vi "Magnetic Drift Correction (1).vi"() -> ()   [LabVIEW 2025]
uses:
  <instrlib>/SMS LabVIEW Drivers/Source Code/Cryogenic Ltd SMSXXX.lvlib
  LabVIEW VI's/Instrument VI's/Instrument Controls/Magnet Array.ctl
  <instrlib>/SMS LabVIEW Drivers/Source Code/Public/PSU Status.ctl
  Labview-File/QMH (STM Auto)/CTL's/Scan_Params (QMH).ctl
  Labview-File/Magnetic Drift Correction/XY_Coords(Final).ctl
panel:
  in  "P-Mode Ramp Rate (A/s)":dbl
  out "Final coordinates (m)":cluster{"Xc":sgl, "Yc":sgl} {"Yc" format="%.4p"; "Xc" format="%.4p"}
  out "Initial coordinates (m)":cluster{"Xc":sgl, "Yc":sgl} {"Yc" format="%.4p"; "Xc" format="%.4p"}
  out "Translation (m)":T1
  out "Output (T)":dbl
  out "MID Setpoint (T)":dbl
  in  "Field Range":T2={"Sweep States"=enum."SET FIELD", "VISA Connection"="COM4", "Fields(T)"=[]}
  in  "Lead- Mode Ramp Rate (A/s)":dbl=0.02
  in  "Start":bool
  out "Errors":errorcluster[](array[cluster])
  in  "stop":bool
  out "Current Index":i32
  in  "Next Field":bool
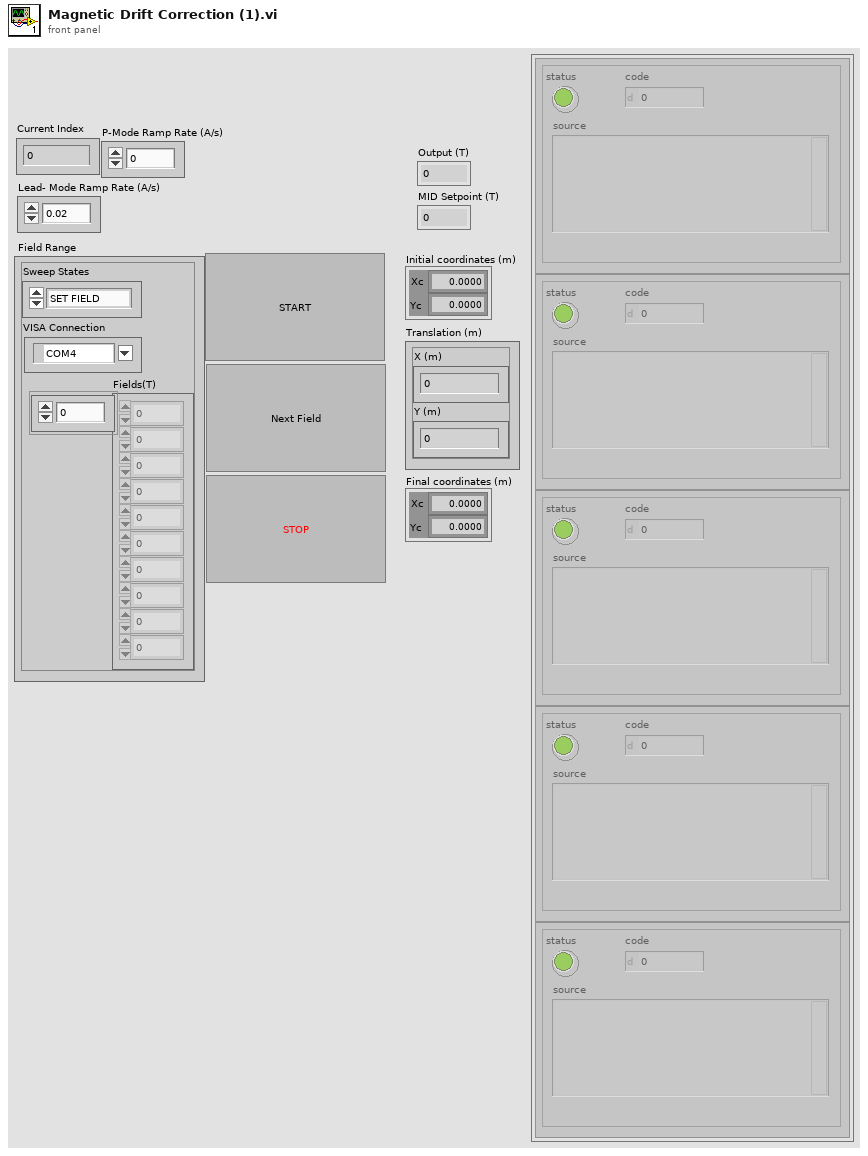
[diagram p1: front panel]
types:
  T1 = typedef "XY_Coords(Final).ctl" = cluster{"X (m)":dbl, "Y (m)":dbl}
  T2 = cluster{"Sweep States":enum16{"SET FIELD", "SWEEP IDLE", "NEXT FIELD", "SWEEP DONE"}, "VISA Connection":refnum<visa-resource-name>, "Fields(T)":dbl[]}
  T3 = enum16{"1. INIT MAG", "2. MAG ON", "3. MAG_STAB", "4. MAG IDLE", "5. PREP NEXT FIELD", "6. APPLY NEXT FIELD", "7. PREP OFF", "8. MAG OFF (Reset)"}
  T4 = typedef "Scan_Params (QMH).ctl" = cluster{"Setpoint (I)":dbl[], "Bias (V)":dbl[], "Number of scans":u8, "Port number (3364)":u32, "Avoid zero threshold (V)":dbl, "Current State":enum16{"1. BIAS", "2. INIT_SCAN", "3. SCAN_IDLE", "4. INTER_SCAN", "5. NEW_COORDS_&_FRAME", "6. FINAL_SCAN", "7. POLL BIAS", "8. Z-CONT", "9. STOP"}}
  T5 = enum16{"1. BIAS", "2. INIT_SCAN", "3. SCAN_IDLE", "4. INTER_SCAN", "5. NEW_COORDS_&_FRAME", "6. FINAL_SCAN", "7. STOP"}
  T6 = typedef "Cryogenic Ltd SMSXXX.lvlib/PSU Status.ctl" = cluster{"Ramp Target":enum16{"ZERO", "MID", "MAX"}, "Pause":bool, "Switch Heater":bool, "Persistent Field":dbl, "Persistent Current":dbl, "Tesla":bool, "Output (T)":dbl, "Output (A)":dbl, "X Trip":enum16{"DISABLED", "ENABLED", "ACTIVE"}, "Ramp Rate (A/s)":dbl, "V Limit (V)":dbl, "Heater Voltage":dbl, "MAX Setpoint (A)":dbl, "MAX Setpoint (T)":dbl, "MID Setpoint (A)":dbl, "MID Setpoint (T)":dbl, "Lock":bool, "Field Constant":dbl, "Remote":bool, "Direction":enum16{"POSITIVE", "NEGATIVE", "OPEN", "UNIPOLAR"}, "Helium Level":u16, "Quench !":bool, "Voltage":dbl, "V Limit !":bool, "Ramping":bool, "At Target":bool, "Trip Field":dbl, "Trip Current":dbl, "Enum":enum16{"1. INIT MAG", "2. MAG ON ", "3. MAG_STAB", "4. MAG IDLE", "5. NEXT FIELD", "6. MAG OFF (Reset)"}}
  T7 = enum16{"SET FIELD", "SWEEP IDLE", "NEXT FIELD", "SWEEP DONE"}
  T8 = typedef "Magnet Array.ctl" = cluster{"Sweep States":enum16{"SET FIELD", "SWEEP IDLE", "NEXT FIELD", "SWEEP DONE"}, "VISA Connection":refnum<visa-resource-name>, "Fields(T)":dbl[]}
  T9 = typedef "Scan_Params (QMH).ctl" = cluster{"Setpoint (I)":dbl[], "Bias (V)":dbl[], "Number of scans":u8, "Port number (3364)":u32, "Avoid zero threshold (V)":dbl, "Current State":enum16{"1. BIAS", "2. INIT_SCAN", "3. SCAN_IDLE", "4. INTER_SCAN", "5. NEW_COORDS_&_FRAME", "6. FINAL_SCAN", "7. POLL BIAS ", "8. STOP"}}
  T10 = enum16{"1. BIAS", "2. INIT_SCAN", "3. SCAN_IDLE", "4. INTER_SCAN", "5. NEW_COORDS_&_FRAME", "6. FINAL_SCAN", "7. POLL BIAS ", "8. STOP"}
  T11 = typedef "Bias Cont QMH.ctl" = cluster{"Machine name (local machine IP)":string, "Port number (3364)":u32, "Current State":enum16{"Bias", "Stop"}, "Inital X (m)":dbl, "Initial Y (m)":dbl, "Final X (m)":sgl, "Final Y (m)":sgl}
  T12 = enum16{"RAMP TO ZERO", "RAMP TO MID", "RAMP TO MAX"}
  T13 = typedef "PSU Status.ctl" = cluster{"Ramp Target":enum16{"ZERO", "MID", "MAX"}, "Pause":bool, "Switch Heater":bool, "Persistent Field":dbl, "Persistent Current":dbl, "Tesla":bool, "Output (T)":dbl, "Output (A)":dbl, "X Trip":enum16{"DISABLED", "ENABLED", "ACTIVE"}, "Ramp Rate (A/s)":dbl, "V Limit (V)":dbl, "Heater Voltage":dbl, "MAX Setpoint (A)":dbl, "MAX Setpoint (T)":dbl, "MID Setpoint (A)":dbl, "MID Setpoint (T)":dbl, "Lock":bool, "Field Constant":dbl, "Remote":bool, "Direction":enum16{"POSITIVE", "NEGATIVE", "OPEN", "UNIPOLAR"}, "Helium Level":u16, "Quench !":bool, "Voltage":dbl, "V Limit !":bool, "Ramping":bool, "At Target":bool, "Trip Field":dbl, "Trip Current":dbl, "Current State":enum16{"1. INIT MAG", "2. MAG ON", "3. MAG_STAB", "4. MAG IDLE", "5. PREP NEXT FIELD", "6. APPLY NEXT FIELD", "7. PREP OFF", "8. MAG OFF (Reset)"}, "MAG Reference":refnum<visa-resource-name>}
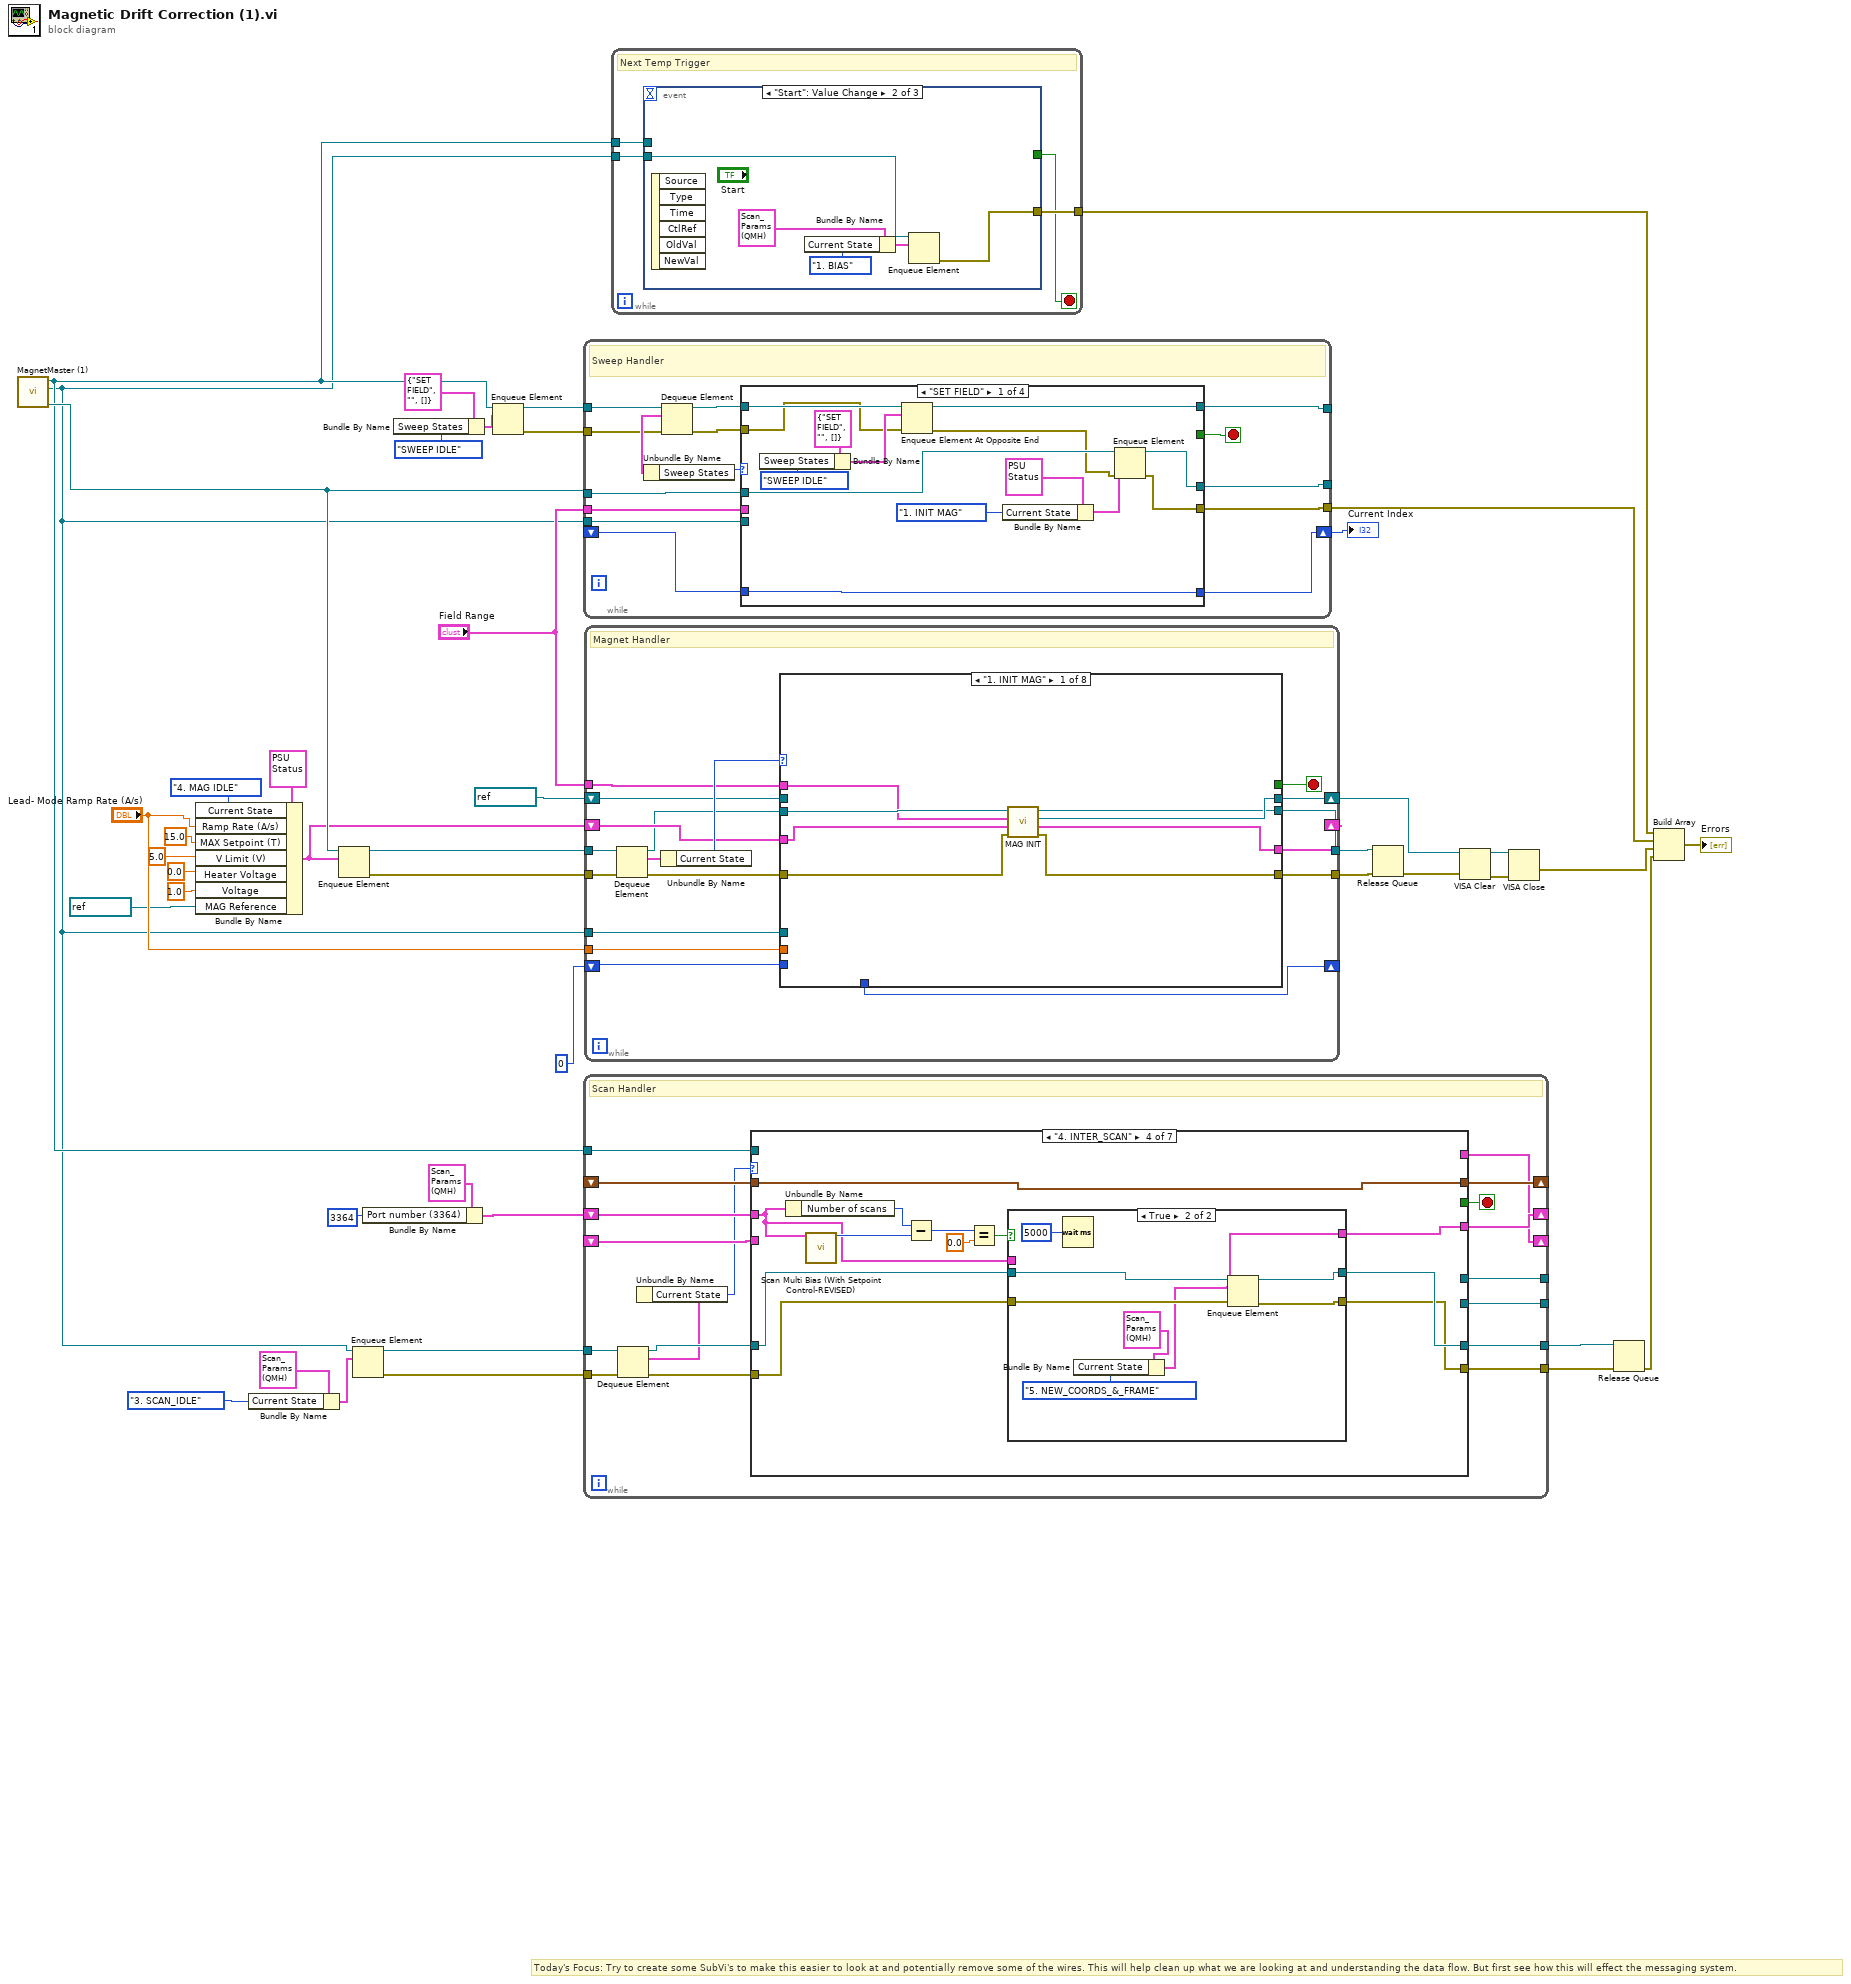
[diagram p0: block diagram]
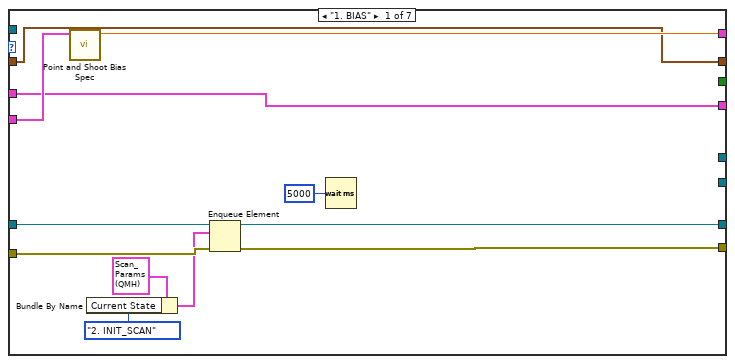
[diagram p2: hidden frame]
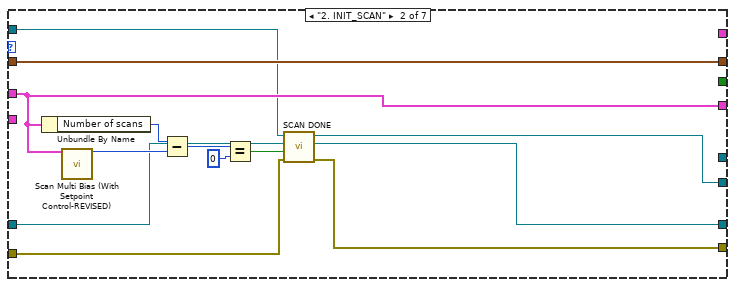
[diagram p3: hidden frame]
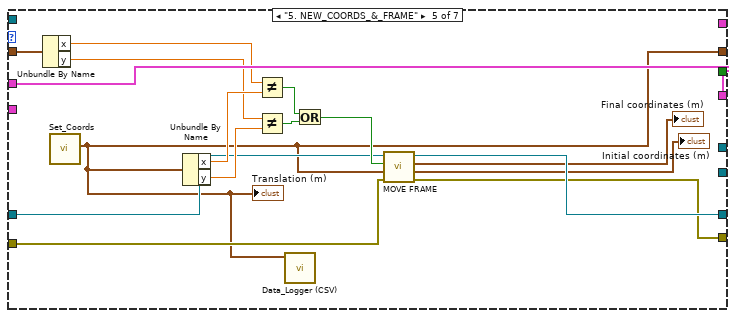
[diagram p6: hidden frame]
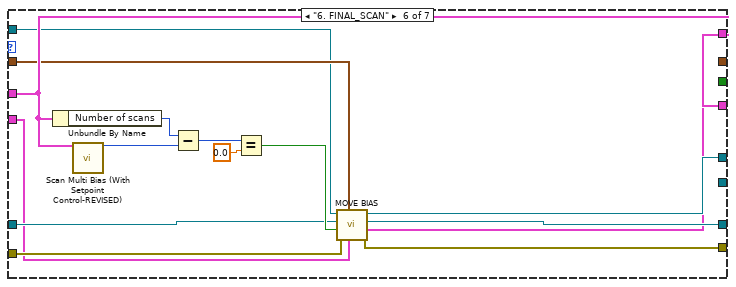
[diagram p7: hidden frame]
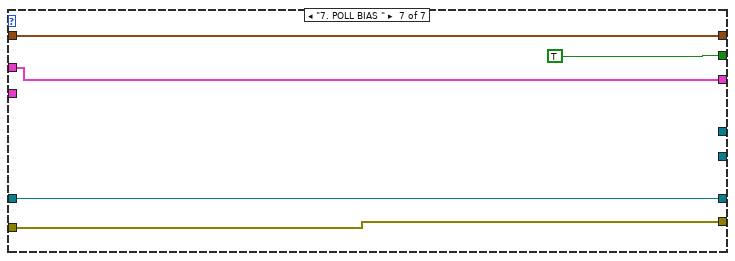
[diagram p8: hidden frame]
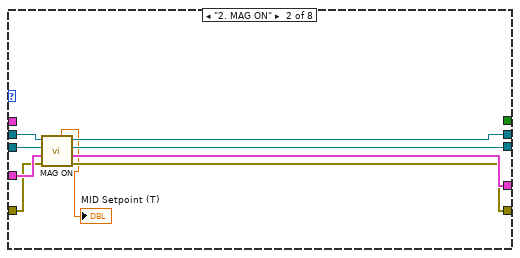
[diagram p9: hidden frame]
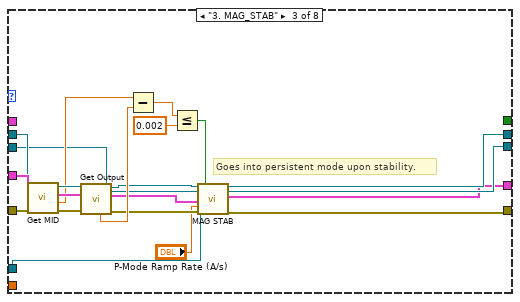
[diagram p10: hidden frame]
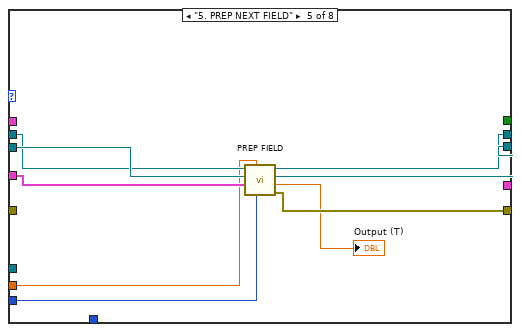
[diagram p12: hidden frame]
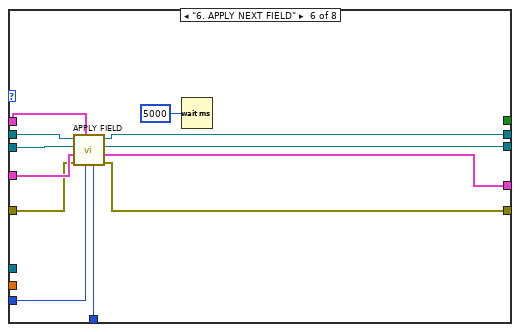
[diagram p13: hidden frame]
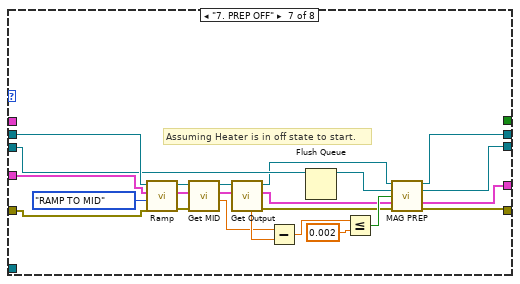
[diagram p14: hidden frame]
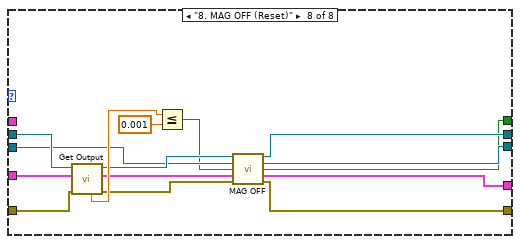
[diagram p15: hidden frame]
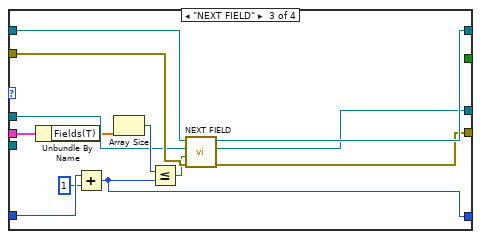
[diagram p17: hidden frame]
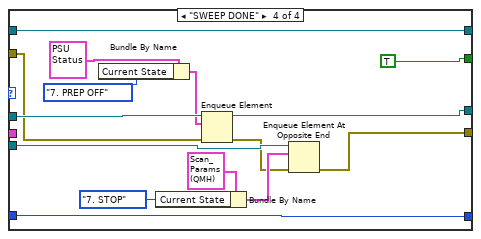
[diagram p18: hidden frame]
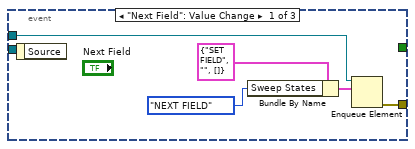
[diagram p19: hidden frame]
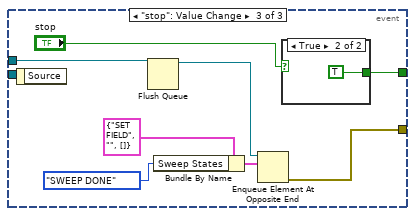
[diagram p20: hidden frame]
diagram:
  # "Today's Focus: Try to create some SubVi's to make this easier to look at and potentially remove some of the wires. This will help clean up what we are looking at and understanding the data flow. But first see how this will effect the messaging system."
  n1 = call "MagnetMaster (1).vi"() -> ("MagQ"=w34:refnum<queue>, "ScanQ"=w1:refnum<queue>, "SweepQ"=w2:refnum<queue>)  [unwired: 9 in]
  n2 = Bundle By Name(cluster=T6 {"Ramp Target"=enum."ZERO", "Pause"=FALSE, "Switch Heater"=FALSE, "Persistent Field"=0.0, "Persistent Current"=0.0, "Tesla"=FALSE, "Output (T)"=0.0, "Output (A)"=0.0, "X Trip"=enum."DISABLED", "Ramp Rate (A/s)"=0.0, "V Limit (V)"=0.0, "Heater Voltage"=0.0, "MAX Setpoint (A)"=0.0, "MAX Setpoint (T)"=0.0, "MID Setpoint (A)"=0.0, "MID Setpoint (T)"=0.0, "Lock"=FALSE, "Field Constant"=0.0, "Remote"=FALSE, "Direction"=enum."POSITIVE", "Helium Level"=0, "Quench !"=FALSE, "Voltage"=0.0, "V Limit !"=FALSE, "Ramping"=FALSE, "At Target"=FALSE, "Trip Field"=0.0, "Trip Current"=0.0, "Enum"=enum."1. INIT MAG"} ("PSU Status In"), "Current State"=T3."4. MAG IDLE", "Ramp Rate (A/s)"="Lead- Mode Ramp Rate (A/s)", "MAX Setpoint (T)"=15.0, "V Limit (V)"=5.0, "Heater Voltage"=0.0, "Voltage"=1.0, "MAG Reference"=refnum<visa-resource-name> "COM4") -> (w30:T6)
  n3 = Bundle By Name(cluster=T4 {"Setpoint (I)"=[], "Bias (V)"=[], "Number of scans"=1, "Port number (3364)"=3364, "Avoid zero threshold (V)"=0.004999999888241291, "Current State"=enum."1. BIAS"} ("element"), "Current State"=T5."3. SCAN_IDLE") -> (w19:T4)
  n4 = Enqueue Element(queue=w34, element=w30) -> (queue out=w33:refnum<queue>, error out=w32:errorcluster)  [unwired: 2 in, 1 out]
  n5 = Enqueue Element(queue=w1, element=w19) -> (queue out=w21:refnum<queue>, error out=w20:errorcluster)  [unwired: 2 in, 1 out]
  n6 = Bundle By Name(cluster=T4 {"Setpoint (I)"=[], "Bias (V)"=[], "Number of scans"=1, "Port number (3364)"=3364, "Avoid zero threshold (V)"=0.004999999888241291, "Current State"=enum."1. BIAS"} ("element"), "Port number (3364)"=u32 3364) -> (w12:T4)
  n7 = Bundle By Name(cluster=T8 {"Sweep States"=enum."SET FIELD", "VISA Connection"="", "Fields(T)"=[]} ("element"), "Sweep States"=T7."SWEEP IDLE") -> (w37:T8)
  n8 = Enqueue Element(queue=w2, element=w37) -> (queue out=w39:refnum<queue>, error out=w35:errorcluster)  [unwired: 2 in, 1 out]
  n9 = while {
    tunnel: w39 -> [w58]
    shift-right: [w53] -> w44
    shift-left: _ -> [w56]
    tunnel: [w55] -> _
    tunnel: [w52] -> _
    tunnel: [w50] -> w28
    tunnel: w34 -> [w48]
    tunnel: w35 -> [w47]
    tunnel: "Field Range" -> [w46]
    tunnel: w1 -> [w45]
    stop <- w49 stop-if-true
    # "Sweep Handler"
    n10 = Dequeue Element(queue=w58, error in (no error)=w47) -> (queue out=w54:refnum<queue>, element=w57:T8, error out=w51:errorcluster)  [unwired: 1 in, 1 out]
    n11 = Unbundle By Name(w57) -> ("Sweep States"=w59:T7)
    n12 = case shown="\"SET FIELD\"" w59 {
      tunnel: w56 -> [w72 _ w86 w100]
      tunnel: [w73 _ w77 w96] -> w55
      tunnel: w54 -> [w71 _ w83 w101]
      tunnel: [w72 _ w76 w100] -> w53
      tunnel: [w70 _ w82 w101] -> w52
      tunnel: w51 -> [w65 _ w81 w97]
      tunnel: [w63 _ w80 w87] -> w50
      tunnel: [_ _ _ TRUE] -> w49
      tunnel: w48 -> [w69 _ w78 w98]
      tunnel: w46 -> [_ _ w74 _]
      tunnel: w45 -> [_ _ _ w91]
      frame "SET FIELD" {
        n13 = Bundle By Name(cluster=T8 {"Sweep States"=enum."SET FIELD", "VISA Connection"="", "Fields(T)"=[]} ("element"), "Sweep States"=T7."SWEEP IDLE") -> (w67:T8)
        n14 = Enqueue Element At Opposite End(queue=w71, element=w67, error in (no error)=w65) -> (queue out=w70:refnum<queue>, error out=w64:errorcluster)  [unwired: 1 in, 1 out]
        n15 = Bundle By Name(cluster=T6 {"Ramp Target"=enum."ZERO", "Pause"=FALSE, "Switch Heater"=FALSE, "Persistent Field"=0.0, "Persistent Current"=0.0, "Tesla"=FALSE, "Output (T)"=0.0, "Output (A)"=0.0, "X Trip"=enum."DISABLED", "Ramp Rate (A/s)"=0.0, "V Limit (V)"=0.0, "Heater Voltage"=0.0, "MAX Setpoint (A)"=0.0, "MAX Setpoint (T)"=0.0, "MID Setpoint (A)"=0.0, "MID Setpoint (T)"=0.0, "Lock"=FALSE, "Field Constant"=0.0, "Remote"=FALSE, "Direction"=enum."POSITIVE", "Helium Level"=0, "Quench !"=FALSE, "Voltage"=0.0, "V Limit !"=FALSE, "Ramping"=FALSE, "At Target"=FALSE, "Trip Field"=0.0, "Trip Current"=0.0, "Enum"=enum."1. INIT MAG"} ("PSU Status In"), "Current State"=T3."1. INIT MAG") -> (w61:T6)
        n16 = Enqueue Element(queue=w69, element=w61, error in (no error)=w64) -> (queue out=w73:refnum<queue>, error out=w63:errorcluster)  [unwired: 1 in, 1 out]
      }
      frame "SWEEP IDLE" {
      }
      frame "NEXT FIELD" {
        n17 = Unbundle By Name(w74) -> ("Fields(T)"=w75:dbl[])
        n18 = Add(x=w86, y=1) -> (x+y=w76:i32)
        n19 = Array Size(array=w75) -> (size(s)=w84:i32)
        n20 = Less Or Equal?(x=w84, y=w76) -> (x <= y?=w79:bool)
        n21 = call "NEXT FIELD.vi"("error in (no error)"=w81, "Boolean"=w79, "MagQ in"=w78, "Queue in"=w83) -> ("error out"=w80:errorcluster, "MagQ out"=w77:refnum<queue>, "Queue out"=w82:refnum<queue>)  [unwired: 5 in]
      }
      frame "SWEEP DONE" {
        n22 = Bundle By Name(cluster=T6 {"Ramp Target"=enum."ZERO", "Pause"=FALSE, "Switch Heater"=FALSE, "Persistent Field"=0.0, "Persistent Current"=0.0, "Tesla"=FALSE, "Output (T)"=0.0, "Output (A)"=0.0, "X Trip"=enum."DISABLED", "Ramp Rate (A/s)"=0.0, "V Limit (V)"=0.0, "Heater Voltage"=0.0, "MAX Setpoint (A)"=0.0, "MAX Setpoint (T)"=0.0, "MID Setpoint (A)"=0.0, "MID Setpoint (T)"=0.0, "Lock"=FALSE, "Field Constant"=0.0, "Remote"=FALSE, "Direction"=enum."POSITIVE", "Helium Level"=0, "Quench !"=FALSE, "Voltage"=0.0, "V Limit !"=FALSE, "Ramping"=FALSE, "At Target"=FALSE, "Trip Field"=0.0, "Trip Current"=0.0, "Enum"=enum."1. INIT MAG"} ("PSU Status In"), "Current State"=T3."7. PREP OFF") -> (w94:T6)
        n23 = Bundle By Name(cluster=T4 {"Setpoint (I)"=[], "Bias (V)"=[], "Number of scans"=1, "Port number (3364)"=3364, "Avoid zero threshold (V)"=0.004999999888241291, "Current State"=enum."1. BIAS"} ("element"), "Current State"=T5."7. STOP") -> (w90:T4)
        n24 = Enqueue Element(queue=w98, element=w94, error in (no error)=w97) -> (queue out=w96:refnum<queue>, error out=w88:errorcluster)  [unwired: 1 in, 1 out]
        n25 = Enqueue Element At Opposite End(queue=w91, element=w90, error in (no error)=w88) -> (error out=w87:errorcluster)  [unwired: 1 in, 2 out]
      }
    }
  }
  "Current Index" <- w44
  n26 = while {
    tunnel: w20 -> [w111]
    shift-right: [w116] -> _
    shift-left: w12 -> [w119]
    tunnel: [w118] -> w16
    shift-right: [w115] -> _
    shift-left: _ -> [w114]
    tunnel: [w112] -> w15
    tunnel: [w109] -> _
    shift-right: [w107] -> _
    shift-left: _ -> [w108]
    tunnel: w21 -> [w106]
    tunnel: w2 -> [w105]
    tunnel: [w104] -> _
    stop <- w113 stop-if-true
    # "Scan Handler"
    n27 = Dequeue Element(queue=w106, error in (no error)=w111) -> (queue out=w117:refnum<queue>, element=w102:T9, error out=w110:errorcluster)  [unwired: 1 in, 1 out]
    n28 = Unbundle By Name(w102) -> ("Current State"=w103:T10)
    n29 = case shown="\"4. INTER_SCAN\"" w103 {
      tunnel: w119 -> [w127 w137 w146 w151 w186 w197 w203]
      tunnel: [w128 w138 w145 w153 w177 w193 w205] -> w118
      tunnel: w110 -> [w123 w140 _ w148 w174 w191 w204]
      tunnel: w117 -> [w129 w139 w145 w154 w178 w195 w205]
      tunnel: [w127 w137 w146 w152 w186 w197 w203] -> w116
      tunnel: [w126 w135 w147 w150 w171 _ w202] -> w115
      tunnel: w114 -> [w126 w135 w147 w150 w176 w194 w202]
      tunnel: [_ _ _ _ _ _ TRUE] -> w113
      tunnel: [w124 w134 _ w149 w175 w192 w204] -> w112
      tunnel: [_ _ _ _ _ w190 _] -> w109
      tunnel: w108 -> [w131 _ _ _ _ w188 _]
      tunnel: [w130 _ _ _ _ w189 _] -> w107
      tunnel: w105 -> [_ w133 _ _ _ w187 _]
      tunnel: [_ w132 _ _ _ _ _] -> w104
      frame "1. BIAS" {
        n30 = call "Point and Shoot Bias Spec.vi"("Bias Controller"=w131) -> ("Inital X (m)"=w130:dbl)  [unwired: 9 in, 1 out]
        n31 = Bundle By Name(cluster=T4 {"Setpoint (I)"=[], "Bias (V)"=[], "Number of scans"=1, "Port number (3364)"=3364, "Avoid zero threshold (V)"=0.004999999888241291, "Current State"=enum."1. BIAS"} ("element"), "Current State"=T5."2. INIT_SCAN") -> (w120:T4)
        n32 = Enqueue Element(queue=w129, element=w120, error in (no error)=w123) -> (queue out=w128:refnum<queue>, error out=w124:errorcluster)  [unwired: 1 in, 1 out]
        n33 = Wait (ms)(milliseconds to wait=u32 5000) -> ()  [unwired: 1 out]
      }
      frame "2. INIT_SCAN" {
        n34 = Unbundle By Name(w137) -> ("Number of scans"=w136:u8)
        n35 = call "Scan Multi Bias (With Setpoint Control-REVISED).vi"("Scan Parameters"=w137) -> ("Scan"=w141:u8)  [unwired: 13 in, 1 out]
        n36 = Subtract(x=w136, y=w141) -> (x-y=w144:u8)
        n37 = Equal?(x=w144, y=u8 0) -> (x = y?=w142:bool)
        n38 = call "SCAN DONE.vi"("error in (no error)"=w140, "Boolean"=w142, "ScanQ in"=w139, "Queue in"=w133) -> ("error out"=w134:errorcluster, "ScanQ out"=w138:refnum<queue>, "Queue out"=w132:refnum<queue>)  [unwired: 5 in]
      }
      frame "3. SCAN_IDLE" {
      }
      frame "4. INTER_SCAN" {
        n39 = Unbundle By Name(w151) -> ("Number of scans"=w155:u8)
        n40 = call "Scan Multi Bias (With Setpoint Control-REVISED).vi"("Scan Parameters"=w151) -> ("Scan"=w156:u8)  [unwired: 13 in, 1 out]
        n41 = Subtract(x=w155, y=w156) -> (x-y=w158:u8)
        n42 = Equal?(x=w158, y=0.0) -> (x = y?=w157:bool)
        n43 = case shown="True" w157 {
          tunnel: w154 -> [w162 w169]
          tunnel: [w162 w168] -> w153
          tunnel: [w161 w163] -> w152
          tunnel: w151 -> [w161 _]
          tunnel: [w160 w167] -> w149
          tunnel: w148 -> [w160 w166]
          frame False {
          }
          frame True {
            n44 = Wait (ms)(milliseconds to wait=u32 5000) -> ()  [unwired: 1 out]
            n45 = Bundle By Name(cluster=T4 {"Setpoint (I)"=[], "Bias (V)"=[], "Number of scans"=1, "Port number (3364)"=3364, "Avoid zero threshold (V)"=0.004999999888241291, "Current State"=enum."2. INIT_SCAN"} ("element"), "Current State"=T5."5. NEW_COORDS_&_FRAME") -> (w163:T4)
            n46 = Enqueue Element(queue=w169, element=w163, error in (no error)=w166) -> (queue out=w168:refnum<queue>, error out=w167:errorcluster)  [unwired: 1 in, 1 out]
          }
        }
      }
      frame "5. NEW_COORDS_&_FRAME" {
        n47 = Unbundle By Name(w176) -> ("x"=w180:dbl, "y"=w179:dbl)
        n48 = call "Set_Coords.vi"() -> ("return value"=w171:cluster{"x":dbl, "y":dbl})  [unwired: 10 in, 1 out]
        "Translation (m)" <- w171
        n49 = Unbundle By Name(w171) -> ("x"=w183:dbl, "y"=w182:dbl)
        n50 = Not Equal?(x=w180, y=w183) -> (x != y?=w185:bool)
        n51 = Not Equal?(x=w179, y=w182) -> (x != y?=w184:bool)
        n52 = call "Data_Logger (CSV).vi"("Translation (m)"=w171) -> ()  [unwired: 11 in]
        n53 = Or(x=w185, y=w184) -> (x .or. y?=w181:bool)
        n54 = call "MOVE FRAME.vi"("error in (no error)"=w174, "return value"=w171, "Boolean"=w181, "Queue in"=w178) -> ("error out"=w175:errorcluster, "Initial coordinates (m)"=→"Initial coordinates (m)":cluster{"Xc":sgl, "Yc":sgl}, "Final coordinates (m)"=→"Final coordinates (m)":cluster{"Xc":sgl, "Yc":sgl}, "Queue out"=w177:refnum<queue>)  [unwired: 4 in]
      }
      frame "6. FINAL_SCAN" {
        n55 = Unbundle By Name(w197) -> ("Number of scans"=w196:u8)
        n56 = call "Scan Multi Bias (With Setpoint Control-REVISED).vi"("Scan Parameters"=w197) -> ("Scan"=w199:u8)  [unwired: 13 in, 1 out]
        n57 = Subtract(x=w196, y=w199) -> (x-y=w200:u8)
        n58 = Equal?(x=w200, y=0.0) -> (x = y?=w198:bool)
        n59 = call "MOVE BIAS.vi"("Bias in"=w188, "return value"=w194, "error in (no error)"=w191, "Boolean"=w198, "ScanQ in"=w195, "Queue in"=w187) -> ("error out"=w192:errorcluster, "Bias out 2"=w189:T11, "ScanQ out"=w193:refnum<queue>, "Queue out"=w190:refnum<queue>)  [unwired: 2 in]
      }
      frame "7. POLL BIAS " {
      }
    }
  }
  n60 = while {
    tunnel: w33 -> [w223]
    tunnel: [w219] -> w42
    shift-right: [w218] -> _
    shift-left: w30 -> [w221]
    shift-right: [w217] -> w8
    shift-left: refnum<visa-resource-name> "COM4" ("MAG Reference") -> [w216]
    tunnel: [w215] -> w43
    tunnel: w32 -> [w214]
    tunnel: "Field Range" -> [w213]
    shift-right: [w208] -> _
    shift-left: 0 -> [w212]
    tunnel: "Lead- Mode Ramp Rate (A/s)" -> [w210]
    tunnel: w1 -> [w209]
    stop <- w207 stop-if-true
    # "Magnet Handler"
    n61 = Dequeue Element(queue=w223, error in (no error)=w214) -> (queue out=w211:refnum<queue>, element=w224:T13, error out=w220:errorcluster)  [unwired: 1 in, 1 out]
    n62 = Unbundle By Name(w224) -> ("Current State"=w222:T3)
    n63 = case "MAG STATE MACHINE" shown="\"1. INIT MAG\"" w222 {
      tunnel: w221 -> [w228 w241 w261 w266 w272 w283 w308 w323]
      tunnel: w220 -> [w226 w239 w262 w265 _ w282 w307 w324]
      tunnel: [w231 w236 w242 w265 w269 w286 w288 w311] -> w219
      tunnel: [w229 w237 w243 w266 _ w278 w289 w314] -> w218
      tunnel: [w232 w238 w246 w264 w268 w279 w291 w315] -> w217
      tunnel: w216 -> [_ w240 w260 w264 w271 w284 w309 w325]
      tunnel: [w230 w235 w247 w263 w274 w287 w290 w313] -> w215
      tunnel: w213 -> [w225 _ _ _ _ w281 _ _]
      tunnel: w212 -> [_ _ _ _ w275 w280 _ _]
      tunnel: w211 -> [w227 w234 w251 w263 w273 w277 w299 w318]
      tunnel: w210 -> [_ _ _ _ w270 _ _ _]
      tunnel: w209 -> [_ _ w250 _ _ _ _ _]
      tunnel: [_ _ _ _ _ w276 _ _] -> w208
      tunnel: [_ _ _ _ _ _ _ w312] -> w207
      frame "1. INIT MAG" {
        n64 = call "MAG INIT.vi"("error in (no error)"=w226, "PSU Status In"=w228, "Field and Temp Range"=w225, "Queue in"=w227) -> ("error out"=w231:errorcluster, "PSU Status Out"=w229:T6, "VISA Resource Name Out"=w232:refnum<visa-resource-name>, "Queue out"=w230:refnum<queue>)  [unwired: 4 in]
      }
      frame "2. MAG ON" {
        n65 = call "MAG ON.vi"("error in (no error)"=w239, "PSU Status In"=w241, "MagQ in"=w234, "VISA Refnum in"=w240) -> ("error out"=w236:errorcluster, "PSU Status Out"=w237:T6, "MagQ out"=w235:refnum<queue>, "VISA Refnum out"=w238:refnum<visa-resource-name>, "MID Setpoint (T)"=→"MID Setpoint (T)":dbl)  [unwired: 3 in]
      }
      frame "3. MAG_STAB" {
        # "Goes into persistent mode upon stability."
        n66 = call <instrlib>:"Get MID.vi"("Error in (no error)"=w262, "PSU Status In"=w261, "VISA Resource Name In"=w260) -> ("Error out"=w259:errorcluster, "MID Setpoint (T)"=w255:dbl, "PSU Status Out"=w258:T6, "VISA Resource Name Out"=w257:refnum<visa-resource-name>)  [unwired: 3 in, 2 out]
        n67 = call <instrlib>:"Get Output.vi"("Error in (no error)"=w259, "PSU Status In"=w258, "VISA Resource Name In"=w257) -> ("Error out"=w248:errorcluster, "PSU Status Out"=w249:T6, "VISA Resource Name Out"=w252:refnum<visa-resource-name>, "Output (T)"=w253:dbl)  [unwired: 3 in, 2 out]
        n68 = Subtract(x=w255, y=w253) -> (x-y=w254:dbl)
        n69 = Less Or Equal?(x=w254, y=0.002) -> (x <= y?=w245:bool)
        n70 = call "MAG STAB.vi"("VISA In"=w252, "MagQ"=w251, "ScanQ"=w250, "PSU Status In"=w249, "P-Mode Ramp Rate (A/s)"="P-Mode Ramp Rate (A/s)", "Error out"=w248, "Boolean"=w245) -> ("VISA Out"=w246:refnum<visa-resource-name>, "MagQ"=w247:refnum<queue>, "PSU Status Out"=w243:T6, "error out"=w242:errorcluster)  [unwired: 9 in]
      }
      frame "4. MAG IDLE" {
      }
      frame "5. PREP NEXT FIELD" {
        n71 = call "PREP FIELD.vi"("Numeric"=w275, "Lead- Mode Ramp Rate (A/s)"=w270, "PSU Status In"=w272, "MagQ in"=w273, "VISA Refnum in"=w271) -> ("error out"=w269:errorcluster, "Output (T)"=→"Output (T)":dbl, "MagQ out"=w274:refnum<queue>, "VISA Refnum out"=w268:refnum<visa-resource-name>)  [unwired: 3 in]
      }
      frame "6. APPLY NEXT FIELD" {
        n72 = call "APPLY FIELD.vi"("Numeric in"=w280, "Field and Tep  Range"=w281, "error in (no error)"=w282, "PSU Status In"=w283, "MagQ in"=w277, "VISA Refnum in"=w284) -> ("error out"=w286:errorcluster, "PSU Status Out"=w278:T6, "MagQ out"=w287:refnum<queue>, "VISA Refnum out"=w279:refnum<visa-resource-name>, "Numeric out"=w276:i32)  [unwired: 1 in]
        n73 = Wait (ms)(milliseconds to wait=u32 5000) -> ()  [unwired: 1 out]
      }
      frame "7. PREP OFF" {
        # "Assuming Heater is in off state to start."
        n74 = call <instrlib>:"Ramp.vi"("Error in (no error)"=w307, "Ramp Target"=T12."RAMP TO MID", "PSU Status In"=w308, "VISA Resource Name In"=w309) -> ("Error out"=w304:errorcluster, "PSU Status Out"=w305:T6, "VISA Resource Name Out"=w306:refnum<visa-resource-name>)  [unwired: 4 in, 1 out]
        n75 = call <instrlib>:"Get MID.vi"("Error in (no error)"=w304, "PSU Status In"=w305, "VISA Resource Name In"=w306) -> ("MID Setpoint (T)"=w297:dbl, "PSU Status Out"=w302:T6, "VISA Resource Name Out"=w303:refnum<visa-resource-name>)  [unwired: 3 in, 3 out]
        n76 = call <instrlib>:"Get Output.vi"("PSU Status In"=w302, "VISA Resource Name In"=w303) -> ("Error out"=w292:errorcluster, "PSU Status Out"=w293:T6, "VISA Resource Name Out"=w295:refnum<visa-resource-name>, "Output (T)"=w298:dbl)  [unwired: 4 in, 2 out]
        n77 = Subtract(x=w297, y=w298) -> (x-y=w301:dbl)
        n78 = Flush Queue(queue=w299) -> (queue out=w296:refnum<queue>)  [unwired: 1 in, 2 out]
        n79 = Less Or Equal?(x=w301, y=0.002) -> (x <= y?=w294:bool)
        n80 = call "MAG PREP.vi"("VISA In"=w295, "MagQ"=w296, "Boolean"=w294, "PSU Status In"=w293, "Error In"=w292) -> ("VISA Out"=w291:refnum<visa-resource-name>, "MagQ"=w290:refnum<queue>, "PSU Status Out"=w289:T6, "error out"=w288:errorcluster)  [unwired: 7 in]
      }
      frame "8. MAG OFF (Reset)" {
        n81 = call <instrlib>:"Get Output.vi"("Error in (no error)"=w324, "PSU Status In"=w323, "VISA Resource Name In"=w325) -> ("Error out"=w317:errorcluster, "PSU Status Out"=w319:T6, "VISA Resource Name Out"=w320:refnum<visa-resource-name>, "Output (T)"=w322:dbl)  [unwired: 3 in, 2 out]
        n82 = Less Or Equal?(x=w322, y=0.001) -> (x <= y?=w316:bool)
        n83 = call "MAG OFF.vi"("VISA Resource Name Out"=w320, "MagQ"=w318, "Boolean"=w316, "PSU Status Out"=w319, "Error out"=w317) -> ("VISA Resource Name Out 2"=w315:refnum<visa-resource-name>, "MagQ 2"=w313:refnum<queue>, "Boolean 2"=w312:bool, "PSU Status Out 2"=w314:T6, "error out"=w311:errorcluster)  [unwired: 6 in]
      }
    }
  }
  n84 = while {
    tunnel: w2 -> [w329]
    tunnel: [w328] -> w29
    tunnel: w1 -> [w326]
    stop <- w327 stop-if-true
    # "Next Temp Trigger"
    n85 = event shown="[1] \"Start\": Value Change" {
      selector: _ -> [_ _ _]
      dyn-events: _ -> [_ _ _]
      timeout: _ -> [_ _ _]
      tunnel: w329 -> [w334 _ w341]
      tunnel: [w333 w339 w344] -> w328
      tunnel: [_ _ w342] -> w327
      tunnel: w326 -> [_ w337 _]
      event "Next Field": Value Change {
        n86 = event-data() -> ()  [unwired: 1 in, 1 out]
        n87 = Bundle By Name(cluster=T8 {"Sweep States"=enum."SET FIELD", "VISA Connection"="", "Fields(T)"=[]} ("element"), "Sweep States"=T7."NEXT FIELD") -> (w331:T8)
        n88 = Enqueue Element(queue=w334, element=w331) -> (error out=w333:errorcluster)  [unwired: 2 in, 2 out]
      }
      event "Start": Value Change {
        n89 = event-data() -> ()  [unwired: 1 in, 6 out]
        n90 = Bundle By Name(cluster=T4 {"Setpoint (I)"=[], "Bias (V)"=[], "Number of scans"=1, "Port number (3364)"=3364, "Avoid zero threshold (V)"=0.004999999888241291, "Current State"=enum."1. BIAS"} ("element"), "Current State"=T5."1. BIAS") -> (w336:T4)
        n91 = Enqueue Element(queue=w337, element=w336) -> (error out=w339:errorcluster)  [unwired: 2 in, 2 out]
      }
      event "stop": Value Change {
        n92 = event-data() -> ()  [unwired: 1 in, 1 out]
        n93 = Flush Queue(queue=w341) -> (queue out=w340:refnum<queue>)  [unwired: 1 in, 2 out]
        n94 = Bundle By Name(cluster=T8 {"Sweep States"=enum."SET FIELD", "VISA Connection"="", "Fields(T)"=[]} ("element"), "Sweep States"=T7."SWEEP DONE") -> (w346:T8)
        n95 = Enqueue Element At Opposite End(queue=w340, element=w346) -> (error out=w344:errorcluster)  [unwired: 2 in, 2 out]
        n96 = case shown="True" "stop" {
          tunnel: [FALSE ("stop 2") TRUE ("stop 2")] -> w342
          frame False {
          }
          frame True {
          }
        }
      }
    }
  }
  n97 = Release Queue(queue=w43, error in (no error)=w42) -> (error out=w7:errorcluster)  [unwired: 1 in, 2 out]
  n98 = VISA Clear(VISA resource name=w8, error in (no error)=w7) -> (VISA resource name out=w6:refnum<visa-resource-name>, error out=w5:errorcluster)
  n99 = VISA Close(VISA resource name=w6, error in (no error)=w5) -> (error out=w41:errorcluster)
  n100 = Release Queue(queue=w16, error in (no error)=w15) -> (error out=w14:errorcluster)  [unwired: 1 in, 2 out]
  n101 = Build Array(w29, w28, w41, w14) -> (→"Errors":errorcluster[])
